vi "Test bed.vi"() -> ()   [LabVIEW 2019]
panel:
  out "internal idle 2 bot":i32
  in  "change state":bool=TRUE
  out "internal idle 1 bot":i32
  out "internal idle 1 top":i32
  in  "Enum":enum16{"Idle  1", "Idle 2"}(ring)
  in  "stop external":bool
  out "external":i32
  out "internal idle 2 top":i32
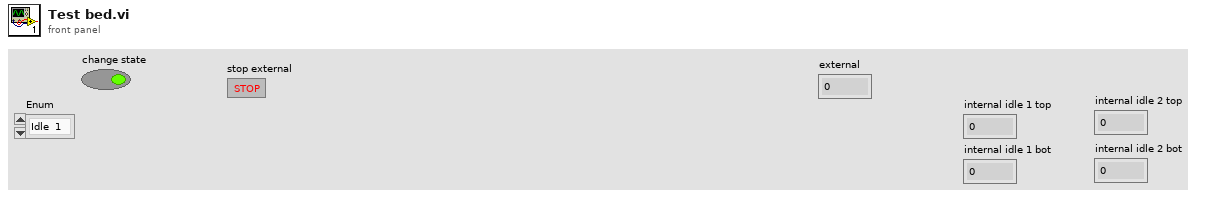
[diagram p1: front panel]
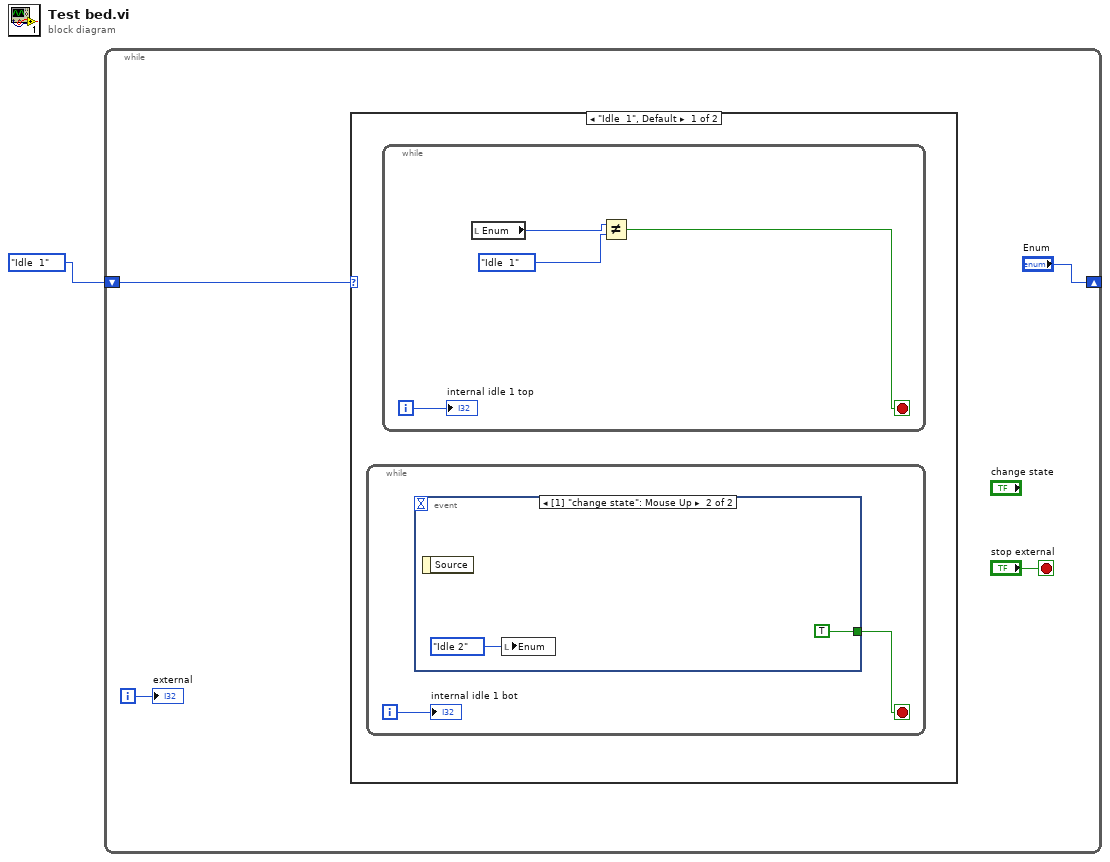
[diagram p0: block diagram]
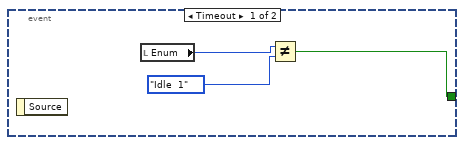
[diagram p2: hidden frame]
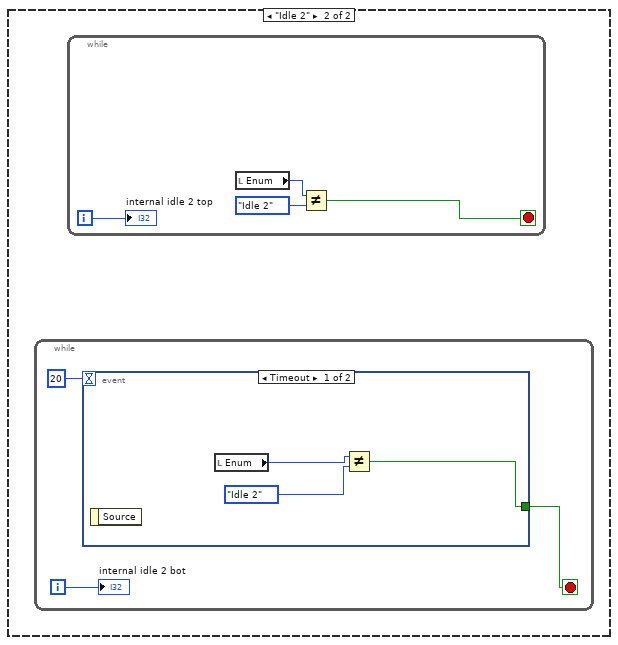
[diagram p3: hidden frame]
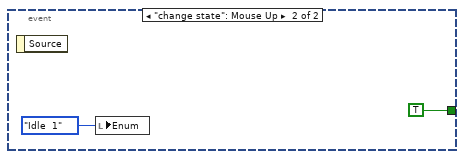
[diagram p4: hidden frame]
diagram:
  n1 = while {
    shift-right: ["Enum"] -> _
    shift-left: enum16{"Idle  1", "Idle 2"}."Idle  1" ("Enum") -> [w3]
    i -> [w4]
    stop <- "stop external" stop-if-true
    n2 = case shown="\"Idle  1\", Default" w3 {
      frame "Idle  1", Default {
        n3 = while {
          i -> [w7]
          stop <- w6 stop-if-true
          n4 = event shown="[1] \"change state\": Mouse Up" {
            selector: _ -> [_ _]
            dyn-events: _ -> [_ _]
            timeout: _ -> [_ _]
            tunnel: [w8 TRUE] -> w6
            event Timeout {
              n5 = event-data() -> ()  [unwired: 1 in, 1 out]
              n6 = local read "Enum"() -> (w10:enum16{"Idle  1", "Idle 2"})
              n7 = Not Equal?(x=w10, y=enum16{"Idle  1", "Idle 2"}."Idle  1" ("Enum")) -> (x != y?=w8:bool)
            }
            event "change state": Mouse Up {
              n8 = event-data() -> ()  [unwired: 1 in, 1 out]
              n9 = local write "Enum"(enum16{"Idle  1", "Idle 2"}."Idle 2" ("Enum")) -> ()
            }
          }
          "internal idle 1 bot" <- w7
        }
        n10 = while {
          i -> [w16]
          stop <- w14 stop-if-true
          n11 = local read "Enum"() -> (w13:enum16{"Idle  1", "Idle 2"})
          n12 = Not Equal?(x=w13, y=enum16{"Idle  1", "Idle 2"}."Idle  1" ("Enum")) -> (x != y?=w14:bool)
          "internal idle 1 top" <- w16
        }
      }
      frame "Idle 2" {
        n13 = while {
          i -> [w19]
          stop <- w18 stop-if-true
          n14 = event shown="[0] Timeout" {
            selector: _ -> [_ _]
            dyn-events: _ -> [_ _]
            timeout: 20 -> [_ _]
            tunnel: [w20 TRUE] -> w18
            event Timeout {
              n15 = event-data() -> ()  [unwired: 1 in, 1 out]
              n16 = local read "Enum"() -> (w22:enum16{"Idle  1", "Idle 2"})
              n17 = Not Equal?(x=w22, y=enum16{"Idle  1", "Idle 2"}."Idle 2" ("Enum")) -> (x != y?=w20:bool)
            }
            event "change state": Mouse Up {
              n18 = event-data() -> ()  [unwired: 1 in, 1 out]
              n19 = local write "Enum"(enum16{"Idle  1", "Idle 2"}."Idle  1" ("Enum")) -> ()
            }
          }
          "internal idle 2 bot" <- w19
        }
        n20 = while {
          i -> [w28]
          stop <- w25 stop-if-true
          n21 = local read "Enum"() -> (w27:enum16{"Idle  1", "Idle 2"})
          n22 = Not Equal?(x=w27, y=enum16{"Idle  1", "Idle 2"}."Idle 2") -> (x != y?=w25:bool)
          "internal idle 2 top" <- w28
        }
      }
    }
    "external" <- w4
  }
